vi "ConfigureSignalTrackEnabled.vi"(8 "error in (no error)":errorcluster, 11 "SpecAnBase in":refnum<class "SpecAnBase.lvclass">) -> (0 "error out":errorcluster, 3 "SpecAnBase out":refnum<class "SpecAnBase.lvclass">)   [LabVIEW 2018, in "SpecAnPlugins.lvlib" / "SpecAnBase.lvclass"]
doc: "This VI turns signal-tracking on/off. When signal tracking is turned on, the spectrum analyzer centers the signal on which the active marker resides after each sweep. There are two prevalent methods of signal tracking in the industry. \n\n1. A search for the largest signal on screen is made, and the spectrum analyzer center frequency is tuned to this signal.\n\n2. The marker is placed on a signal (anywhere on screen) and when marker track is enabled, the frequency of the peak of the selected signal is used for tuning the spectrum analyzer. This does not need to be the largest signal on screen, and this method tracks the specified signal in the presence of a larger signal.\n\nThis VI implements the first method of signal tracking. This INVALIDATES the Frequency Start and Frequency Stop property values. \n\nNote: Signal track can only be enabled on one marker at a time. The driver shall check all other markers to see if this VI is already enabled on any marker other than the active and turn this off on the other marker before enabling this on the active marker."
uses:
  SpecAnBase.lvclass
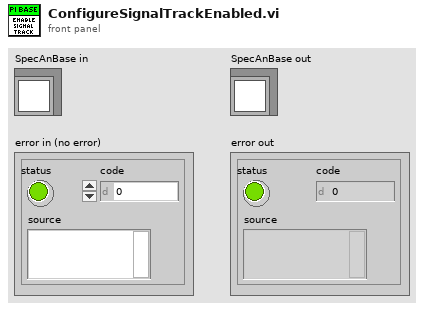
[diagram p1: front panel]
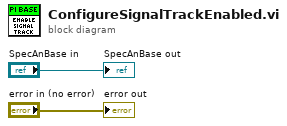
[diagram p0: block diagram]
diagram:
  "error out" <- "error in (no error)"
  "SpecAnBase out" <- "SpecAnBase in"
